vi "Apply.vi"(8 "error in":errorcluster, 11 "Red-y Read Write CFG in":refnum<class "Red-y Pressure Control CFG.lvclass">) -> (0 "error out":errorcluster, 3 "Red-y Read Write CFG out":refnum<class "Red-y Pressure Control CFG.lvclass">)   [LabVIEW 2023, in "Red-y Pressure Control CFG.lvclass"]
uses:
  Red-y Pressure Control CFG.lvclass
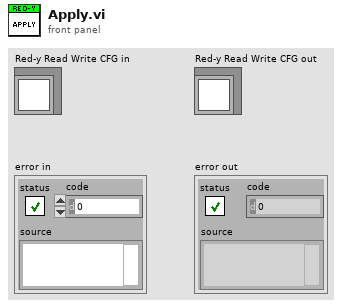
[diagram p1: front panel]
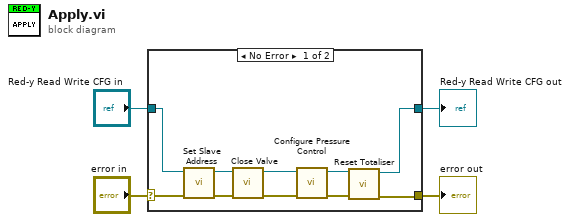
[diagram p0: block diagram]
diagram:
  n1 = case shown="No Error" "error in" {
    selector: "error in" -> [w14 w16]
    tunnel: [w6 w16] -> w3
    tunnel: [w5 w15] -> w1
    tunnel: "Red-y Read Write CFG in" -> [w12 w15]
    frame No Error {
      n2 = call-dynamic "Set Slave Address.vi"("error in"=w14, "Red-y Read Write CFG in"=w12) -> ("error out"=w13:errorcluster, "Red-y Read Write CFG out"=w10:refnum<class "Red-y Pressure Control CFG.lvclass">)  [unwired: 8 in]
      n3 = call-dynamic "Close Valve.vi"("error in"=w13, "Red-y Read Write CFG in"=w10) -> ("error out"=w11:errorcluster, "Red-y Read Write CFG out"=w9:refnum<class "Red-y Pressure Control CFG.lvclass">)  [unwired: 8 in]
      n4 = call-dynamic "Configure Pressure Control.vi"("error in"=w11, "Red-y Read Write CFG in"=w9) -> ("error out"=w7:errorcluster, "Red-y Read Write CFG out"=w8:refnum<class "Red-y Pressure Control CFG.lvclass">)  [unwired: 8 in]
      n5 = call-dynamic "Reset Totaliser.vi"("error in"=w7, "Red-y Read Write CFG in"=w8) -> ("error out"=w6:errorcluster, "Red-y Read Write CFG out"=w5:refnum<class "Red-y Pressure Control CFG.lvclass">)  [unwired: 8 in]
    }
    frame Error {
    }
  }
  "error out" <- w3
  "Red-y Read Write CFG out" <- w1
